vi "DI NO.vi"(11 "DI no 1":u16) -> (3 "DI no 1 Out":u16)   [LabVIEW 2014]
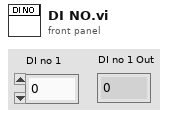
[diagram p1: front panel]
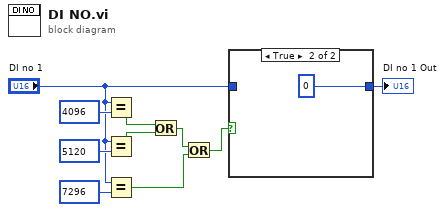
[diagram p0: block diagram]
diagram:
  n1 = Equal?(x="DI no 1", y=u16 4096) -> (x = y?=w8:bool)
  n2 = Equal?(x="DI no 1", y=u16 5120) -> (x = y?=w7:bool)
  n3 = Equal?(x="DI no 1", y=u16 7296) -> (x = y?=w2:bool)
  n4 = Or(x=w8, y=w7) -> (x .or. y?=w5:bool)
  n5 = Or(x=w5, y=w2) -> (x .or. y?=w4:bool)
  n6 = case shown="True" w4 {
    tunnel: "DI no 1" -> [w11 _]
    tunnel: [w11 u16 0 ("DI no 1")] -> w6
    frame False {
    }
    frame True {
    }
  }
  "DI no 1 Out" <- w6
